vi "ATSpectrograph_issueCommand_changeFilter.vi"(8 "error in (no error)":errorcluster, 11 "command_changeFilter_Ctl":T1) -> (0 "error out":errorcluster, 2 "function return":i32, 3 "command_changeFilter_Ctl out":T1)   [LabVIEW 2016, in "SALLV_ATSpectrograph.lvlib"]
doc: "int ATSpectrograph_shm_issueCommand_changeFilterLV(ATSpectrograph_command_changeFilterLV *command_changeFilter_Ctl );"
uses:
  SALLV_ATSpectrograph.lvlib
  DataTypes/command_changeFilter.ctl
  SALLV_ATSpectrograph.so
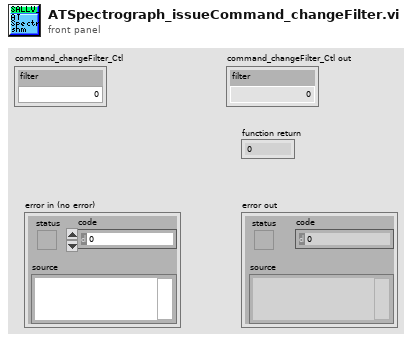
[diagram p1: front panel]
types:
  T1 = typedef "SALLV_ATSpectrograph.lvlib/command_changeFilter.ctl" = cluster{"filter":i32}
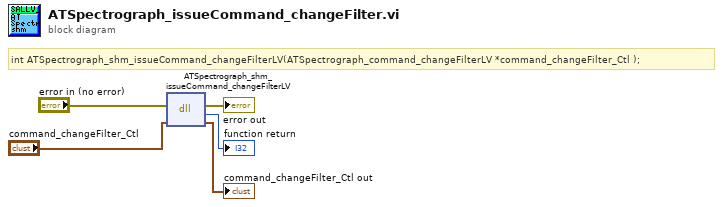
[diagram p0: block diagram]
diagram:
  # "int ATSpectrograph_shm_issueCommand_changeFilterLV(ATSpectrograph_command_changeFilterLV *command_changeFilter_Ctl );"
  n1 = dll-call lib="home/harini/tcs/SALLV_ATSpectrograph/SALLV_ATSpectrograph.*" fn="ATSpectrograph_shm_issueCommand_changeFilterLV"(error in="error in (no error)", "command_changeFilter_Ctl"="command_changeFilter_Ctl") -> (error out=→"error out":errorcluster, →"function return":i32, "command_changeFilter_Ctl"=→"command_changeFilter_Ctl out":T1)  [unwired: 2 in, 1 out]
